vi "bubble sort subnodes.vi"(7 "Sort by":T1, 9 "subnodes category in":string[](array[string]), 10 "subnodes class in":string[](array[string]), 11 "subnodes menu name in":string[](array[string])) -> (1 "subnodes category out":string[](array[string]), 2 "subnodes class out":string[](array[string]), 3 "subnodes menu name out":string[](array[string]))   [LabVIEW 2013, in "PL Framework Configuration Tool.lvlib" / "Engine Parent Editor Node.lvclass"]
uses:
  Engine Parent Editor Node.lvclass
  subnodes sort by.ctl
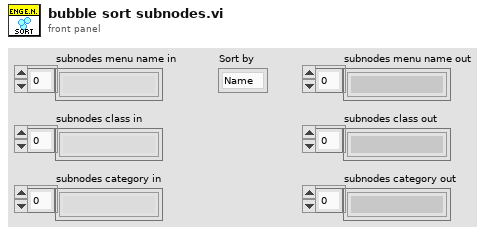
[diagram p1: front panel]
types:
  T1 = typedef "PL Framework Configuration Tool.lvlib/Engine Parent Editor Node.lvclass/subnodes sort by.ctl" = enum16{"Name", "Class", "Category"}
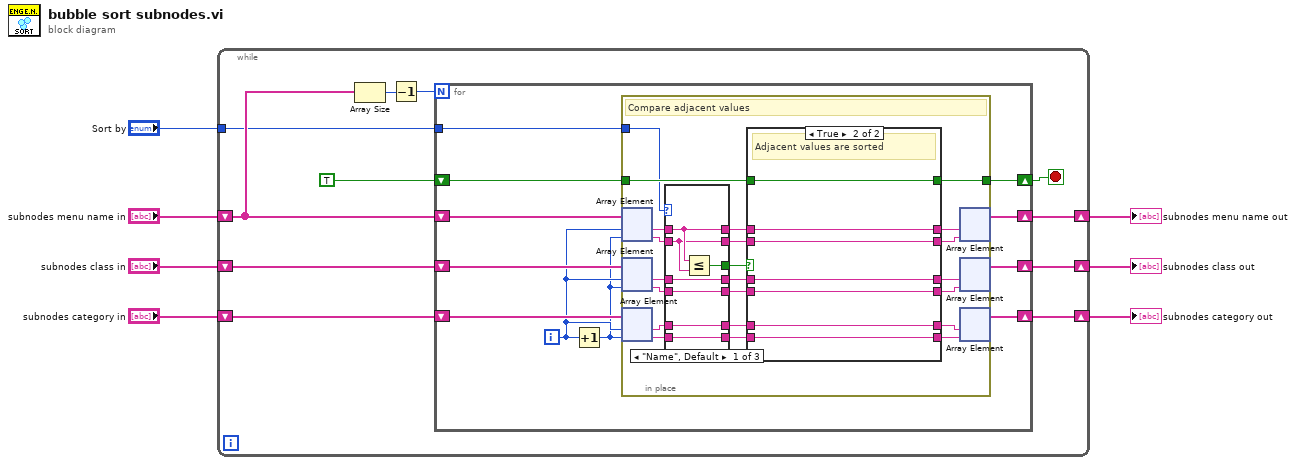
[diagram p0: block diagram]
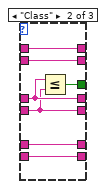
[diagram p2: hidden frame]
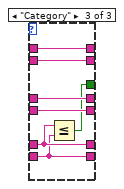
[diagram p3: hidden frame]
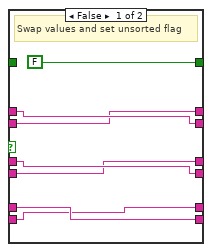
[diagram p4: hidden frame]
diagram:
  n1 = while {
    shift-right: [w17] -> w1
    shift-left: "subnodes menu name in" -> [w18]
    shift-right: [w10] -> w6
    shift-left: "subnodes class in" -> [w12]
    shift-right: [w9] -> w7
    shift-left: "subnodes category in" -> [w11]
    tunnel: "Sort by" -> [w8]
    stop <- w13 stop-if-true
    n2 = Array Size(array=w18) -> (size(s)=w14:i32)
    n3 = Decrement(x=w14) -> (x-1=w15:i32)
    n4 = for {
      N: w15 -> [_]
      shift-right: [w28] -> w17
      shift-left: w18 -> [w29]
      shift-right: [w26] -> w13
      shift-left: TRUE -> [w27]
      shift-right: [w21] -> w10
      shift-left: w12 -> [w25]
      shift-right: [w20] -> w9
      shift-left: w11 -> [w24]
      tunnel: w8 -> [w19]
      i -> [w23]
      n5 = Increment(x=w23) -> (x+1=w22:i32)
      n6 = in-place {
        in-place-border: w27 -> [w48]
        in-place-border: [w47] -> w26
        in-place-border: w19 -> [w42]
        # "Compare adjacent values"
        n7 = in-place-array #1(w29, w23, w22) -> (w41:string, w39:string)
        n8 = in-place-array #2(w25, w23, w22) -> (w36:string, w34:string)
        n9 = in-place-array #3(w24, w23, w22) -> (w32:string, w30:string)
        n10 = case shown="\"Name\", Default" w42 {
          tunnel: [w58 w61 w68] -> w51
          tunnel: w41 -> [w57 w65 w72]
          tunnel: [w57 w65 w72] -> w40
          tunnel: w39 -> [w56 w64 w71]
          tunnel: [w56 w64 w71] -> w38
          tunnel: [w55 w60 w70] -> w37
          tunnel: w36 -> [w55 w60 w70]
          tunnel: [w54 w59 w69] -> w35
          tunnel: w34 -> [w54 w59 w69]
          tunnel: [w53 w63 w67] -> w33
          tunnel: w32 -> [w53 w63 w67]
          tunnel: [w52 w62 w66] -> w31
          tunnel: w30 -> [w52 w62 w66]
          frame "Name", Default {
            n11 = Less Or Equal?(x=w57, y=w56) -> (x <= y?=w58:bool)
          }
          frame "Class" {
            n12 = Less Or Equal?(x=w60, y=w59) -> (x <= y?=w61:bool)
          }
          frame "Category" {
            n13 = Less Or Equal?(x=w67, y=w66) -> (x <= y?=w68:bool)
          }
        }
        n14 = case shown="True" w51 {
          tunnel: [w79 w84] -> w50
          tunnel: w40 -> [w79 w85]
          tunnel: [w77 w85] -> w49
          tunnel: w38 -> [w77 w84]
          tunnel: w48 -> [_ w86]
          tunnel: [FALSE w86] -> w47
          tunnel: [w75 w83] -> w46
          tunnel: w37 -> [w76 w83]
          tunnel: [w76 w82] -> w45
          tunnel: w35 -> [w75 w82]
          tunnel: [w73 w81] -> w44
          tunnel: w33 -> [w74 w81]
          tunnel: [w74 w80] -> w43
          tunnel: w31 -> [w73 w80]
          frame False {
            # "Swap values and set unsorted flag"
          }
          frame True {
            # "Adjacent values are sorted"
          }
        }
        n15 = in-place-array #1(w49, w50) -> (w28:string[])  [unwired: 2 out]
        n16 = in-place-array #2(w46, w45) -> (w21:string[])  [unwired: 2 out]
        n17 = in-place-array #3(w44, w43) -> (w20:string[])  [unwired: 2 out]
      }
    }
  }
  "subnodes category out" <- w7
  "subnodes class out" <- w6
  "subnodes menu name out" <- w1
